vi "Forward Message.vi"(8 "error in (no error)":errorcluster, 9 "Message":string, 10 "Dest Enqueuer":refnum<class "Message Enqueuer.lvclass">, 11 "Connection Listener in":refnum<class "Connection Listener.lvclass">) -> (0 "error out":errorcluster, 3 "Connection Listener out":refnum<class "Connection Listener.lvclass">)   [LabVIEW 2017, in "Connection Listener.lvlib" / "Connection Listener.lvclass"]
uses:
  Connection Listener.lvclass
  C:/Program Files (x86)/National Instruments/LabVIEW 2017/vi.lib/ActorFramework/Actor/Actor.lvclass
  <vilib>/ActorFramework/Message Enqueuer/Message Enqueuer.lvclass
  Connection Listener.lvclass/Connection Listener.ctl
  Connection Handler/Connection Handler Messages/Send Message Msg/Send Message Msg.lvclass/Send Message Msg.ctl
  <vilib>/ActorFramework/Message Enqueuer/Message Enqueuer.lvclass/Message Enqueuer.ctl
  Classes/Message Interface/Status/Status.lvclass
  C:/Users/Public/Documents/wc/BuildFarm/src/LabVIEW/vi.lib/BenjaminR/Build Farm/Classes/Message Interface/iMessage/iMessage.lvclass
  <vilib>/ActorFramework/Actor/Actor.lvclass/Actor.ctl
  Connection Listener Messages/Update UI Msg/Update UI Msg.lvclass/Update UI Msg.ctl
  <vilib>/ActorFramework/Message Enqueuer/Enqueue.vi
  <vilib>/ActorFramework/Message Enqueuer/Init from Existing Queue.vi
  Connection Handler/Connection Handler Messages/Send Message Msg/Send Message Msg.lvclass
  C:/Program Files (x86)/National Instruments/LabVIEW 2017/vi.lib/ActorFramework/Message/Message.lvclass
  Connection Listener Messages/Update UI Msg/Update UI Msg.lvclass
  <vilib>/ActorFramework/Message Priority Queue/Priority Enqueue.vi
  <vilib>/ActorFramework/Actor/Actor.lvclass
  Classes/Message Interface/iMessage/iMessage.lvclass
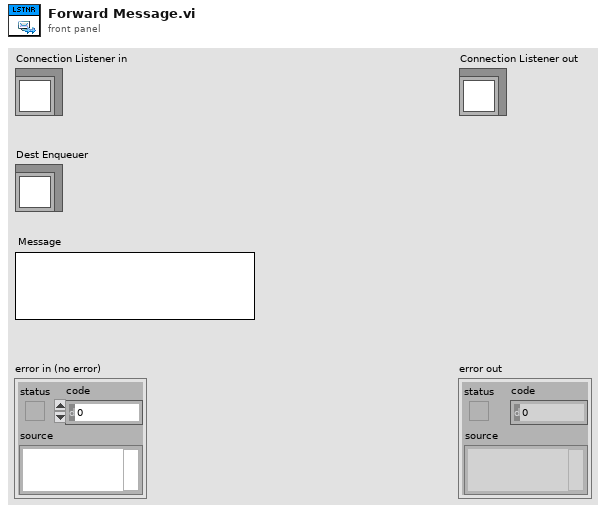
[diagram p1: front panel]
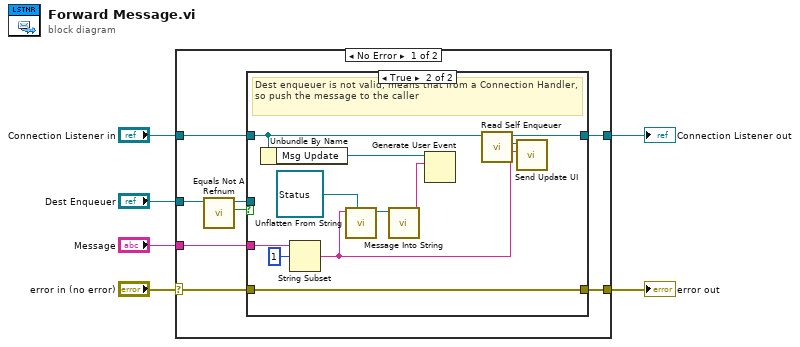
[diagram p0: block diagram]
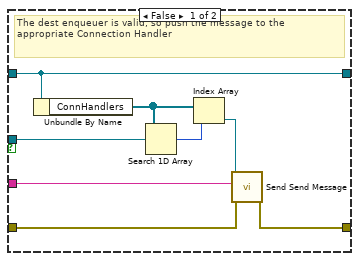
[diagram p2: hidden frame]
diagram:
  n1 = case shown="No Error" "error in (no error)" {
    selector: "error in (no error)" -> [w9 w33]
    tunnel: [w8 w33] -> w5
    tunnel: [w10 w32] -> w3
    tunnel: "Connection Listener in" -> [w11 w32]
    tunnel: "Dest Enqueuer" -> [w12 _]
    tunnel: "Message" -> [w7 _]
    frame No Error {
      n2 = call <vilib>:"Equals Not A Refnum.vi"("Message Enqueuer"=w12) -> ("Not a refnum?"=w13:bool)  [unwired: 10 in]
      n3 = case shown="True" w13 {
        tunnel: w12 -> [w20 _]
        tunnel: w11 -> [w21 w29]
        tunnel: [w21 w29] -> w10
        tunnel: w7 -> [w17 w23]
        tunnel: w9 -> [w15 w31]
        tunnel: [w14 w31] -> w8
        frame False {
          # "The dest enqueuer is valid, so push the message to the appropriate Connection Handler"
          n4 = Unbundle By Name(w21) -> ("ConnHandlers"=w19:refnum<class "Message Enqueuer.lvclass">[])
          n5 = Search 1D Array(1D array=w19, element=w20) -> (index of element=w18:i32)  [unwired: 1 in]
          n6 = Index Array(array=w19, index=w18) -> (element=w16:refnum<class "Message Enqueuer.lvclass">)
          n7 = call "Send Send Message.vi"("error in (no error)"=w15, "Message"=w17, "Message Enqueuer in"=w16) -> ("error out"=w14:errorcluster)  [unwired: 7 in, 1 out]
        }
        frame True {
          # "Dest enqueuer is not valid, means that from a Connection Handler, so push the message to the caller"
          n8 = Unbundle By Name(w29) -> ("Msg Update"=w28:refnum<user-event>)
          n9 = String Subset(string=w23, offset (0)=1) -> (substring=w24:string)  [unwired: 1 in]
          n10 = call "Unflatten From String.vi"("iMessage in"=refnum<class "Status.lvclass"> refnum ("Message Interface.lvlib:Status.lvclass"), "binary string"=w24) -> ("iMessage out"=w27:refnum<class "Status.lvclass">)  [unwired: 8 in, 1 out]
          n11 = call "Message Into String.vi"("iMessage in"=w27) -> ("String"=w22:string)  [unwired: 8 in, 2 out]
          n12 = Generate User Event(user event=w28, event data cluster=w22) -> ()  [unwired: 2 in, 2 out]
          n13 = call <vilib>:"Read Self Enqueuer.vi"("Actor"=w29) -> ("Self Enqueuer"=w30:refnum<class "Message Enqueuer.lvclass">)  [unwired: 10 in]
          n14 = call "Send Update UI.vi"("string"=w24, "Message Enqueuer in"=w30) -> ()  [unwired: 8 in, 2 out]
        }
      }
    }
    frame Error {
    }
  }
  "error out" <- w5
  "Connection Listener out" <- w3
